vi "Execute Hokuyo Command.vi"(8 "error in (no error)":errorcluster, 9 "milliseconds to wait":u32=200, 10 "Hokuyo Command Parameter":T1={"Device Command"="VV", "String Characters"="VV"}, 11 "VISA Refnum in":refnum<visa-resource-name>) -> (0 "error out":errorcluster, 2 "Line Feed Separated Response":string[](array[string]), 3 "VISA Refnum out":refnum<visa-resource-name>)   [LabVIEW 2018]
doc: "This VI takes a <b>Hokuyo Command Parameter</b> type definition and encapsulates the conversion of the parameters into a compatible 'Hokuyo Data' command string, writing the data to the device serial buffers, and interpreting the device response using the NI-VISA drivers."
uses:
  Type Definitions/Hokuyo Command Parameter.ctl
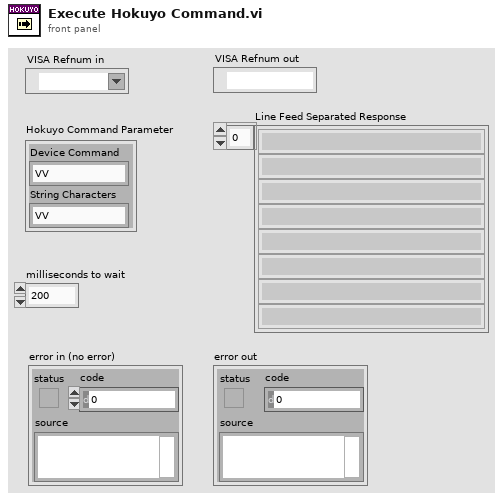
[diagram p1: front panel]
types:
  T1 = typedef "Hokuyo Command Parameter.ctl" = cluster{"Device Command":string, "String Characters":string}
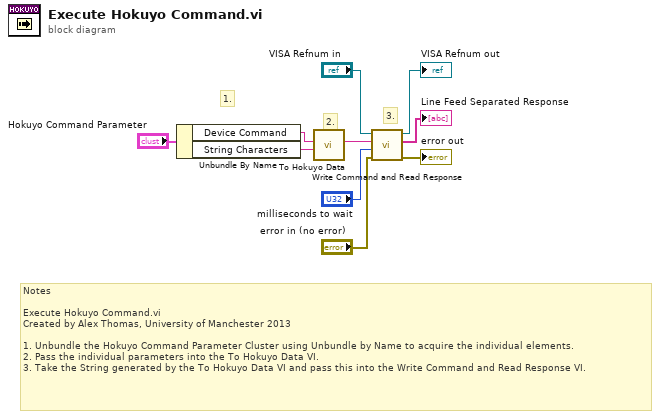
[diagram p0: block diagram]
diagram:
  # "3."
  # "2."
  # "1."
  # "Notes\n\nExecute Hokuyo Command.vi\nCreated by Alex Thomas, University of Manchester 2013\n\n1. Unbundle the Hokuyo Command Parameter Cluster using Unbundle by Name to acquire the individual elements. \n2. Pass the individual parameters into the To Hokuyo Data VI.\n3. Take the String generated by the To Hokuyo Data VI and pass this into the Write Command and Read Response VI."
  n1 = Unbundle By Name("Hokuyo Command Parameter") -> ("Device Command"=w3:string, "String Characters"=w2:string)
  n2 = call "To Hokuyo Data.vi"("String Characters"=w2, "Serial Command"=w3) -> ("Command String"=w6:string)  [unwired: 9 in]
  n3 = call "Write Command and Read Response.vi"("error in (no error)"="error in (no error)", "milliseconds to wait"="milliseconds to wait", "Serial Command"=w6, "VISA Refnum in"="VISA Refnum in") -> ("error out"=→"error out":errorcluster, "Line Feed Separated Response"=→"Line Feed Separated Response":string[], "VISA Refnum out"=→"VISA Refnum out":refnum<visa-resource-name>)  [unwired: 5 in]
